vi "2 Tap 24-Bit RGB.vi"() -> (0 "Pixels":cluster{"Pixel 0":u32, "Pixel 1":u32})   [LabVIEW 2014]
uses:
  <vilib>/rvi/eio/common/nirviEmuTemplateMethod_errors.vi
  <vilib>/eio/EIONode/EIONode.xnode
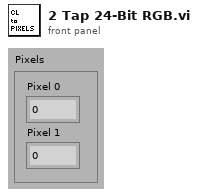
[diagram p1: front panel]
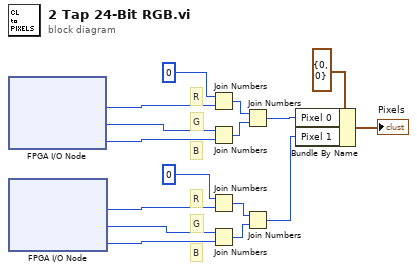
[diagram p0: block diagram]
diagram:
  # "B"
  # "G"
  # "R"
  # "B"
  # "G"
  # "R"
  n1 = xnode "FPGA I/O Node"() -> ("CL Port A"=w12:u8, "CL Port B"=w13:u8, "CL Port C"=w14:u8)  [unwired: 3 in, 3 out]
  n2 = xnode "FPGA I/O Node"() -> ("CL Port D"=w6:u8, "CL Port E"=w7:u8, "CL Port F"=w8:u8)  [unwired: 3 in, 3 out]
  n3 = Join Numbers(hi=u8 0, lo=w12) -> ((hi.lo)=w9:u16)
  n4 = Join Numbers(hi=w13, lo=w14) -> ((hi.lo)=w10:u16)
  n5 = Join Numbers(hi=u8 0, lo=w6) -> ((hi.lo)=w3:u16)
  n6 = Join Numbers(hi=w7, lo=w8) -> ((hi.lo)=w4:u16)
  n7 = Join Numbers(hi=w9, lo=w10) -> ((hi.lo)=w2:u32)
  n8 = Join Numbers(hi=w3, lo=w4) -> ((hi.lo)=w1:u32)
  n9 = Bundle By Name(cluster=cluster{"Pixel 0":u32, "Pixel 1":u32} {"Pixel 0"=0, "Pixel 1"=0} ("PixelData"), "Pixel 0"=w2, "Pixel 1"=w1) -> (→"Pixels":cluster{"Pixel 0":u32, "Pixel 1":u32})
